vi "Get Attribute STRING.vi"(8 "error in":errorcluster, 10 "Attribute":string, 11 "ConfigFromJSON in":refnum<class "Config from JSON.lvclass">) -> (0 "error out":errorcluster, 2 "Value":string, 3 "ConfigFromJSON out":refnum<class "Config from JSON.lvclass">)   [LabVIEW 2024, in "Config from JSON.lvclass"]
uses:
  Config from JSON.lvclass
  <vilib>/JDP Science/JSONtext/LVClass Serializer/JSONtext LVClass Serializer.lvclass
  Config from JSON.lvclass/Config from JSON.ctl
  a5fc0a22-9412-4c72-bc2c-3da30c51af4e.vi
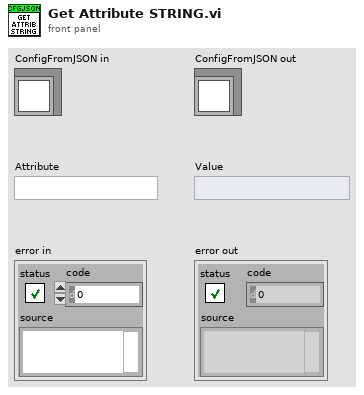
[diagram p1: front panel]
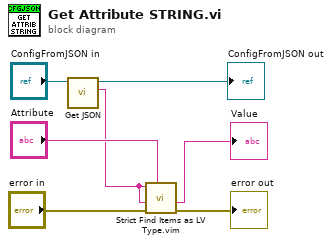
[diagram p0: block diagram]
diagram:
  n1 = call-dynamic "Get JSON.vi"("ConfigFromJSON in"="ConfigFromJSON in") -> ("<JSON>"=w1:string, "ConfigFromJSON out"=→"ConfigFromJSON out":refnum<class "Config from JSON.lvclass">)  [unwired: 9 in]
  n2 = call "Strict Find Items as LV Type.vim"("$Path or Item Name"="Attribute", "error in"="error in", "Data Type and Default Value"=w1, "<JSON>"=w1) -> ("error out"=→"error out":errorcluster, "Data out"=→"Value":string)  [unwired: 6 in]
